vi "Excel_Chart_Font.vi"(0 "axes in":refnum<k7>, 1 "number format":string, 5 "type":i32(ring)=1 items=["xlCategory"=1, "xlSeriesAxis"=3, "xlValue"=2], 11 "error in (no error)":errorcluster, 12 "axis font":T1={"font style"="", "bold"=FALSE, "italic"=FALSE, "underline"=FALSE, "size"=10.0, "color"=-16777216} {"color" items=["wdColorAutomatic"=-16777216, "wdColorBlack"=0, "wdColorBlue"=16711680, "wdColorTurquoise"=16776960, "wdColorBrightGreen"=65280, "wdColorPink"=16711935, "wdColorRed"=255, "wdColorYellow"=65535, "wdColorWhite"=16777215, "wdColorDarkBlue"=8388608, "wdColorTeal"=8421376, "wdColorGreen"=32768, "wdColorViolet"=8388736, "wdColorDarkRed"=128, "wdColorDarkYellow"=32896, "wdColorBrown"=13209, "wdColorOliveGreen"=13107, "wdColorDarkGreen"=13056, "wdColorDarkTeal"=6697728, "wdColorIndigo"=10040115, "wdColorOrange"=26367, "wdColorBlueGray"=10053222, "wdColorLightOrange"=39423, "wdColorLime"=52377, "wdColorSeaGreen"=6723891, "wdColorAqua"=13421619, "wdColorLightBlue"=16737843, "wdColorGold"=52479, "wdColorSkyBlue"=16763904, "wdColorPlum"=6697881, "wdColorRose"=13408767, "wdColorTan"=10079487, "wdColorLightYellow"=10092543, "wdColorLightGreen"=13434828, "wdColorLightTurquoise"=16777164, "wdColorPaleBlue"=16764057, "wdColorLavender"=16751052, "wdColorGray05"=15987699, "wdColorGray10"=15132390, "wdColorGray125"=14737632, "wdColorGray15"=14277081, "wdColorGray20"=13421772, "wdColorGray25"=12632256, "wdColorGray30"=11776947, "wdColorGray35"=10921638, "wdColorGray375"=10526880, "wdColorGray40"=10066329, "wdColorGray45"=9211020, "wdColorGray50"=8421504, "wdColorGray55"=7566195, "wdColorGray60"=6710886, "wdColorGray625"=6316128, "wdColorGray65"=5855577, "wdColorGray70"=5000268, "wdColorGray75"=4210752, "wdColorGray80"=3355443, "wdColorGray85"=2500134, "wdColorGray875"=2105376, "wdColorGray90"=1644825, "wdColorGray95"=789516]; "size" format="%0.2f"}, 13 "title":string) -> (4 "axes out":refnum<k7>, 15 "error out":errorcluster)   [LabVIEW 2020, in "NI_ReportGenerationToolkit.lvlib"]
uses:
  <vilib>/addons/_office/NI_ReportGenerationToolkit.lvlib
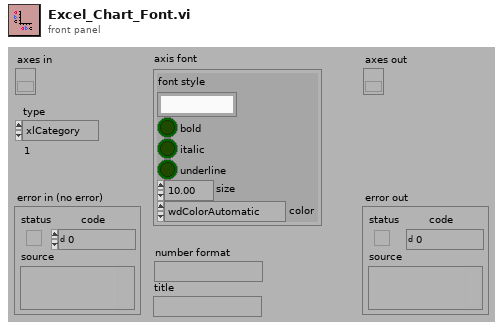
[diagram p1: front panel]
types:
  T1 = cluster{"font style":string, "bold":bool, "italic":bool, "underline":bool, "size":sgl, "color":i32}
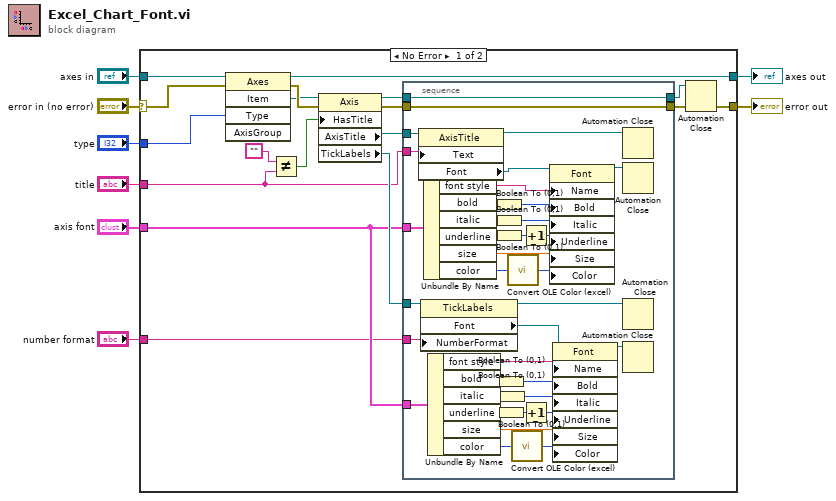
[diagram p0: block diagram]
diagram:
  n1 = case shown="No Error" "error in (no error)" {
    selector: "error in (no error)" -> [w13 w63]
    tunnel: [w26 w64] -> w8
    tunnel: "axes in" -> [w25 w64]
    tunnel: [w14 w63] -> w6
    tunnel: "title" -> [w12 _]
    tunnel: "axis font" -> [w11 _]
    tunnel: "number format" -> [w10 _]
    tunnel: "type" -> [w9 _]
    frame No Error {
      n2 = invoke class="Axes" method="Item"(reference=w25, error in=w13, "Type"=w9) -> (reference out=w26:refnum<k7>, error out=w24:errorcluster, "Item"=w23:refnum<k7>)  [unwired: 2 in, 2 out]
      n3 = Not Equal?(x="", y=w12) -> (x != y?=w17:bool)
      n4 = property class="Axis"(reference=w23, error in=w24, "HasTitle"=w17) -> (reference out=w22:refnum<k7>, error out=w20:errorcluster, "AxisTitle"=w16:refnum<k7>, "TickLabels"=w15:refnum<k7>)
      n5 = stacked-sequence {
        tunnel: w22 -> [w61]
        tunnel: [w61] -> w21
        tunnel: w20 -> [w62]
        tunnel: [w62] -> w19
        tunnel: w16 -> [w60]
        tunnel: w15 -> [w58]
        tunnel: w11 -> [w56]
        tunnel: w11 -> [w55]
        tunnel: w12 -> [w37]
        tunnel: w10 -> [w29]
        frame #0 {
          n6 = property class="AxisTitle"(reference=w60, "Text"=w37) -> (reference out=w36:refnum<k7>, "Font"=w59:refnum<k7>)  [unwired: 1 in, 1 out]
          n7 = property class="TickLabels"(reference=w58, "NumberFormat"=w29) -> (reference out=w34:refnum<k7>, "Font"=w57:refnum<k7>)  [unwired: 1 in, 1 out]
          n8 = Unbundle By Name(w56) -> ("font style"=w51:string, "bold"=w54:bool, "italic"=w53:bool, "underline"=w52:bool, "size"=w47:sgl, "color"=w46:i32)
          n9 = Unbundle By Name(w55) -> ("font style"=w45:string, "bold"=w44:bool, "italic"=w42:bool, "underline"=w40:bool, "size"=w39:sgl, "color"=w38:i32)
          n10 = Boolean To (0,1)(Boolean=w54) -> (0, 1=w50:i16)
          n11 = Boolean To (0,1)(Boolean=w53) -> (0, 1=w49:i16)
          n12 = Boolean To (0,1)(Boolean=w52) -> (0, 1=w48:i16)
          n13 = Boolean To (0,1)(Boolean=w44) -> (0, 1=w43:i16)
          n14 = Boolean To (0,1)(Boolean=w40) -> (0, 1=w32:i16)
          n15 = Boolean To (0,1)(Boolean=w42) -> (0, 1=w41:i16)
          n16 = call <vilib>:"Convert OLE Color (excel).vi"("color in"=w46) -> ("color out"=w27:u32)
          n17 = call <vilib>:"Convert OLE Color (excel).vi"("color in"=w38) -> ("color out"=w28:u32)
          n18 = Increment(x=w48) -> (x+1=w31:i16)
          n19 = Increment(x=w32) -> (x+1=w30:i16)
          n20 = property class="Font"(reference=w59, "Name"=w51, "Bold"=w50, "Italic"=w49, "Underline"=w31, "Size"=w47, "Color"=w27) -> (reference out=w35:refnum<k7>)  [unwired: 1 in, 1 out]
          n21 = property class="Font"(reference=w57, "Name"=w45, "Bold"=w43, "Italic"=w41, "Underline"=w30, "Size"=w39, "Color"=w28) -> (reference out=w33:refnum<k7>)  [unwired: 1 in, 1 out]
          n22 = Automation Close(5:w36) -> ()  [unwired: 1 in, 1 out]
          n23 = Automation Close(5:w35) -> ()  [unwired: 1 in, 1 out]
          n24 = Automation Close(5:w34) -> ()  [unwired: 1 in, 1 out]
          n25 = Automation Close(5:w33) -> ()  [unwired: 1 in, 1 out]
        }
      }
      n26 = Automation Close(3:w19, 5:w21) -> (0:w14:errorcluster)
    }
    frame Error {
    }
  }
  "error out" <- w6
  "axes out" <- w8
